vi "Get Interface.vi"(11 "Transceiver Thread in":refnum<class "Plugin Thread.lvclass">) -> (2 "Interface":refnum<class "Plugin Interface.lvclass">, 3 "Transceiver Thread out":refnum<class "Plugin Thread.lvclass">)   [LabVIEW 2019, in "DSF Core.lvlib" / "Plugin Thread.lvclass"]
uses:
  Thread/Plugin/Plugin Thread.lvclass
  Interface/Plugin/Plugin Interface.lvclass
  Thread/Plugin/Plugin Thread.lvclass/Plugin Thread.ctl
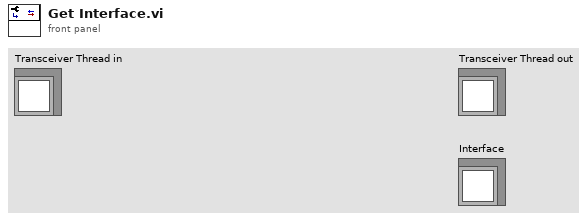
[diagram p1: front panel]
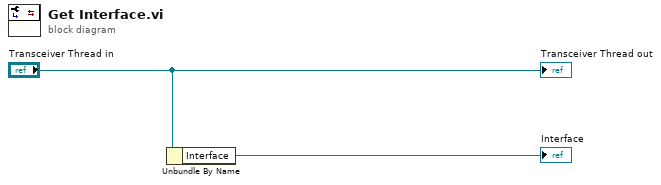
[diagram p0: block diagram]
diagram:
  n1 = Unbundle By Name("Transceiver Thread in") -> ("Interface"=→"Interface":refnum<class "Plugin Interface.lvclass">)
  "Transceiver Thread out" <- "Transceiver Thread in"
